vi "set_name.vi"(8 "error in (no error)":errorcluster, 10 "name":string, 11 "command in":refnum<class "command_generic.lvclass">) -> (0 "error out":errorcluster, 3 "command out":refnum<class "command_generic.lvclass">)   [LabVIEW 2015, in "command_generic.lvclass"]
uses:
  command_generic.lvclass
  command_generic.lvclass/command_generic.ctl
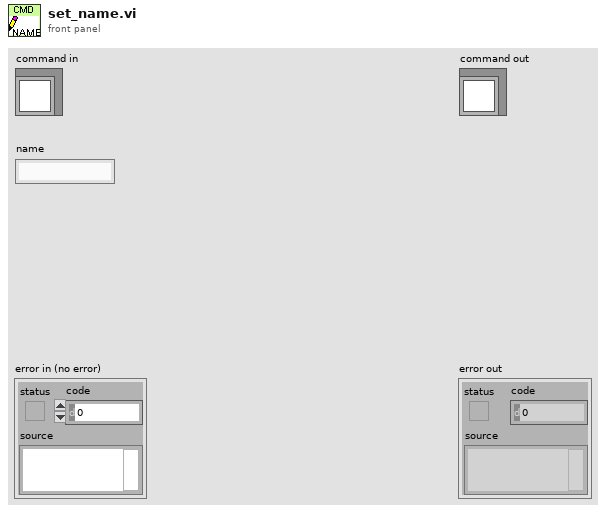
[diagram p1: front panel]
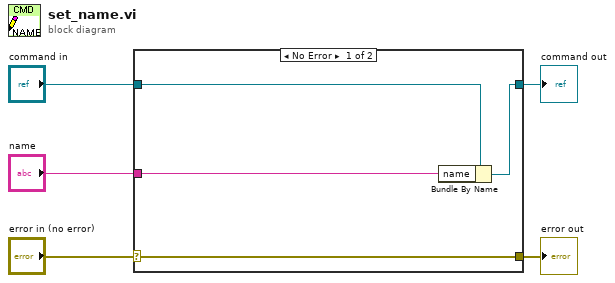
[diagram p0: block diagram]
diagram:
  n1 = case shown="No Error" "error in (no error)" {
    selector: "error in (no error)" -> [w9 w10]
    tunnel: [w9 w10] -> w4
    tunnel: [w7 w11] -> w2
    tunnel: "command in" -> [w8 w11]
    tunnel: "name" -> [w6 _]
    frame No Error {
      n2 = Bundle By Name(cluster=w8, "name"=w6) -> (w7:refnum<class "command_generic.lvclass">)
    }
    frame Error {
    }
  }
  "error out" <- w4
  "command out" <- w2
